vi "Close File+.vi"(0 "error in (no error)":errorcluster, 1 "close when? (now:T)":bool=TRUE, 4 "refnum":refnum<file>) -> (3 "error out":errorcluster, 6 "file size (bytes)":i32, 7 "refnum":refnum<file>)   [LabVIEW 2013]
doc: "Closes the file on command or when an incoming error occurs and returns the file size at closure.\n\nrefnum is the reference number of the open file.\n\nclose when? Set TRUE (default) when you want to close the file when this VI is called. Set to FALSE when you want to close the file only if this VI encounters an incoming error. This input is useful when you use this VI inside a loop and want to close the file only on the last loop iteration or on an upstream error. In that case, set close when? TRUE on the last iteration, and terminate the loop on the last iteration or when this VI returns an error. \n\nfile size is the size of the file in bytes at the time the file is closed; the value is zero otherwise.\n\nerror in is a cluster of three elements (error?, code, and source) that describe the upstream error state, that is, the existence of any error preceding the execution of the VI. The VI executes normally only if no incoming error exists; otherwise it merely passes the error in value to error out. error? is TRUE if an error occurred; the default value is FALSE. code is the error code; the default value is 0. source is in most cases the name of the VI or function that produced the error; the default value is an empty string.\n\ndup refnum is a flow-though parameter with the same value as refnum.\n\nerror out is a cluster of three elements (error?, code, and source) that describe the error state following the execution of the VI. If an incoming error does not exist, the VI executes normally and error out describes the VI's error state; if an incoming error exists, error out equals error in."
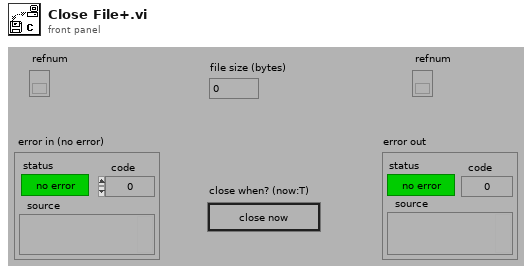
[diagram p1: front panel]
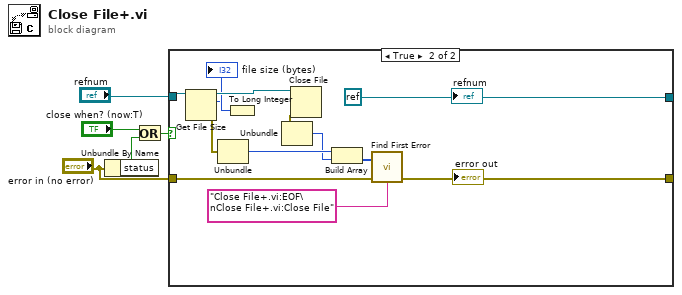
[diagram p0: block diagram]
diagram:
  n1 = Unbundle By Name("error in (no error)") -> ("status"=w1:bool)
  n2 = Or(x="close when? (now:T)", y=w1) -> (x .or. y?=w6:bool)
  n3 = case shown="True" w6 {
    tunnel: [w9 w13] -> w5
    tunnel: "error in (no error)" -> [w9 w16]
    tunnel: [w8 refnum<k0> refnum] -> w4
    tunnel: "refnum" -> [w8 w20]
    frame False {
      # "no incoming error exists and mode is FALSE;\ntherefore, do not close"
    }
    frame True {
      n4 = Get File Size(file=w20) -> (refnum out=w21:refnum<file>, size (in bytes)=w10:i64, 0:w18:errorcluster)  [unwired: 1 in]
      n5 = Unbundle(w18) -> ("code"=w12:i32)  [unwired: 2 out]
      n6 = To Long Integer(number=w10) -> (32bit integer=→"file size (bytes)":i32)
      n7 = Close File(refnum=w21) -> (error out=w17:errorcluster)  [unwired: 1 in, 1 out]
      n8 = Unbundle(w17) -> ("code"=w11:i32)  [unwired: 2 out]
      n9 = Build Array(w12, w11) -> (w15:i32[])
      n10 = call "Find First Error.vi"("error in (no error)"=w16, "source messages"="Close File+.vi:EOF\nClose File+.vi:Close File", "error codes"=w15) -> ("error out"=w13:errorcluster)  [unwired: 1 in, 1 out]
    }
  }
  "error out" <- w5
  "refnum" <- w4
